vi "ChangeComboDeviceNames.vi"(7 "DeviceTypeName":string, 10 "index":i32, 11 "ColumnSetup in":T1[](array[typedef]) {"MinWidth" min=2 step=1; "AutoSizeMode" items=["None"=1, "ColumnHeader"=2, "AllCellsExceptHeader"=4, "AllCells"=6, "DisplayedCellsExceptHeader"=8, "DisplayedCells"=10, "Fill"=16]; "FillWeight" min=1 max=100}) -> (2 "empty?":bool, 3 "ColumnSetup out":T1[](array[typedef]) {"MinWidth" min=2 step=1; "AutoSizeMode" items=["None"=1, "ColumnHeader"=2, "AllCellsExceptHeader"=4, "AllCells"=6, "DisplayedCellsExceptHeader"=8, "DisplayedCells"=10, "Fill"=16]; "FillWeight" min=1 max=100})   [LabVIEW 2013]
uses:
  Shared/LabVIEWdotNetDataGrid-master/source/GridColumn/ColumnDefinition.ctl
  Shared/LabVIEWdotNetDataGrid-master/source/GridColumn/ColumnType.ctl
  Shared/LabVIEWdotNetDataGrid-master/source/GridColumn/GridColumn.lvclass
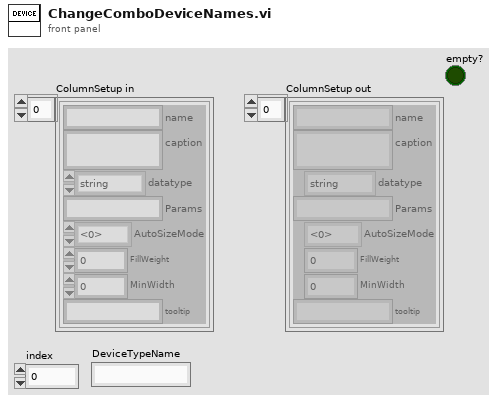
[diagram p1: front panel]
types:
  T1 = typedef "DataGrid.lvlib/GridColumn.lvclass/ColumnDefinition.ctl" = cluster{"name":string, "caption":string, "datatype":T2, "Params":string, "AutoSizeMode":i32, "FillWeight":sgl, "MinWidth":u32, "tooltip":string}
  T2 = typedef "DataGrid.lvlib/GridColumn.lvclass/ColumnType.ctl" = enum16{"string", "image", "check", "numeric", "timestamp", "button", "combo", "link"}
  T3 = typedef "mysql_authentication.ctl" = cluster{"User":string, "Password":string, "Database":string}
  T4 = cluster{"Port":u16, "IP Address":string, "Authentication":T3}
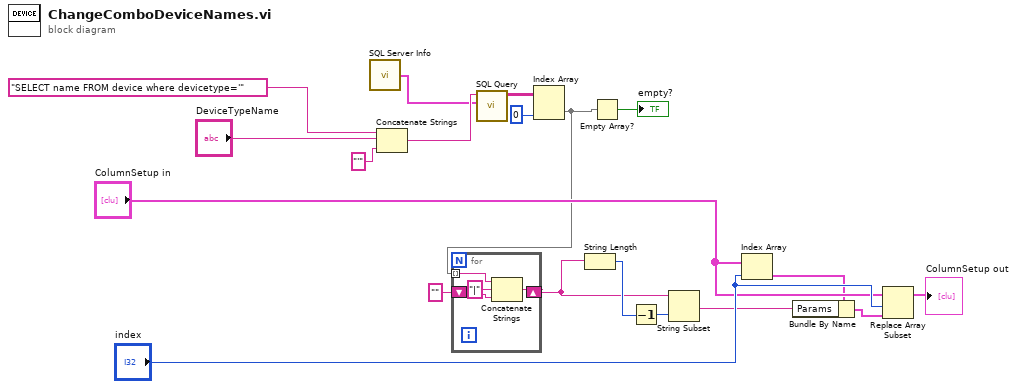
[diagram p0: block diagram]
diagram:
  n1 = call "SQL Server Info.vi"() -> ("SQL Server Info"=w4:T4)
  n2 = Concatenate Strings("SELECT name FROM device where devicetype='" ("Query"), "DeviceTypeName", "'" ("string")) -> (w9:string)
  n3 = call "SQL Query.vi"("SQL Server Info"=w4, "Query"=w9) -> ("data"=w5:string[][])  [unwired: 8 in, 1 out]
  n4 = Index Array(array=w5, index (col)=0 ("disabled index (col)")) -> (element=w2:string[])  [unwired: 1 in]
  n5 = for {
    tunnel: w2 -> [w23] mode=indexing
    shift-right: [w21] -> w12
    shift-left: "" -> [w20]
    n6 = Concatenate Strings(w23, "|" ("string"), w20) -> (w21:string)
  }
  n7 = String Length(string=w12) -> (length=w13:i32)
  n8 = Empty Array?(array=w2) -> (empty?=→"empty?":bool)
  n9 = Decrement(x=w13) -> (x-1=w11:i32)
  n10 = String Subset(string=w12, length (rest)=w11) -> (substring=w15:string)  [unwired: 1 in]
  n11 = Index Array(array="ColumnSetup in", index="index") -> (element=w14:T1)
  n12 = Bundle By Name(cluster=w14, "Params"=w15) -> (w17:T1)
  n13 = Replace Array Subset(array="ColumnSetup in", new element=w17, index="index") -> (→"ColumnSetup out":T1[])
